vi "Initialize DLL Readers.vi"(8 "error in (no error)":errorcluster, 10 "Poll Timeout [5 ms]":i32=5, 11 "Phasor Data Concentrator in":refnum<class "Phasor Data Concentrator.lvclass">) -> (0 "error out":errorcluster, 3 "Phasor Data Concentrator out":refnum<class "Phasor Data Concentrator.lvclass">)   [LabVIEW 2013, in "PMU Recorder Light.lvlib" / "Phasor Data Concentrator.lvclass"]
uses:
  Phasor Data Concentrator.lvclass
  Phasor Data Concentrator.lvclass/Phasor Data Concentrator.ctl
  PMU Recorder Light.lvlib
  Statnett C37.118 DLL/Statnett C37.118 DLL.lvclass
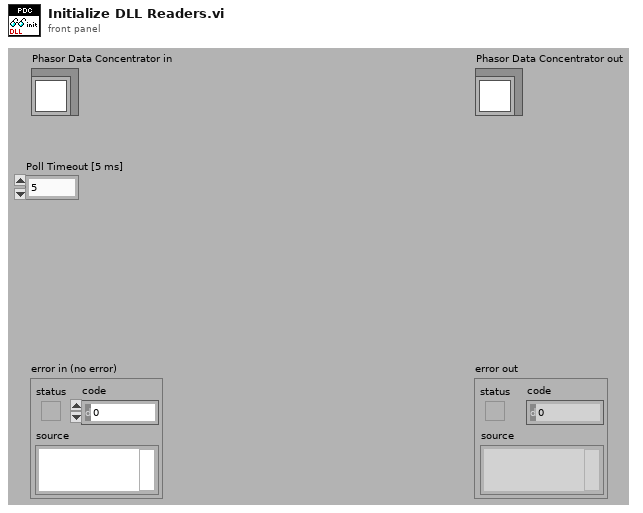
[diagram p1: front panel]
types:
  T1 = cluster{"Phasor":string[], "Analog":string[], "Digital":string[]}
  T2 = cluster{"Pseudo PDC ID":i32, cluster{i32, i32, i32}}
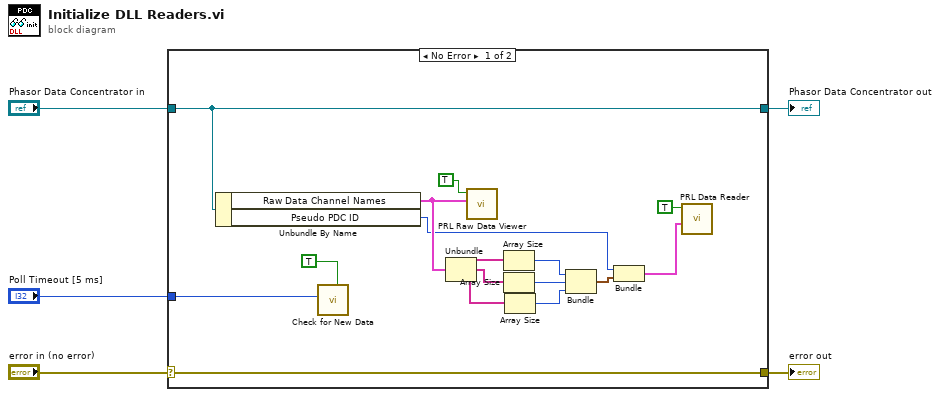
[diagram p0: block diagram]
diagram:
  n1 = case shown="No Error" "error in (no error)" {
    selector: "error in (no error)" -> [w21 w23]
    tunnel: [w21 w23] -> w4
    tunnel: [w20 w22] -> w2
    tunnel: "Phasor Data Concentrator in" -> [w20 w22]
    tunnel: "Poll Timeout [5 ms]" -> [w6 _]
    frame No Error {
      n2 = Unbundle By Name(w20) -> ("Raw Data Channel Names"=w17:T1, "Pseudo PDC ID"=w9:i32)
      n3 = call "Check for New Data.vi"("Set Timeout"=TRUE, "Poll Timeout [5 ms]"=w6) -> ()  [unwired: 8 in, 2 out]
      n4 = Unbundle(w17) -> ("Phasor"=w16:string[], "Analog"=w15:string[], "Digital"=w14:string[])
      n5 = call "PRL Raw Data Viewer.vi"("Raw Data Channel Names"=w17, "Initialize"=TRUE) -> ()  [unwired: 10 in]
      n6 = Array Size(array=w16) -> (size(s)=w13:i32)
      n7 = Array Size(array=w15) -> (size(s)=w12:i32)
      n8 = Array Size(array=w14) -> (size(s)=w11:i32)
      n9 = Bundle(w13, w12, w11) -> (w10:cluster{i32, i32, i32})  [unwired: 1 in]
      n10 = Bundle("Pseudo PDC ID"=w9, w10) -> (w8:T2)  [unwired: 1 in]
      n11 = call "PRL Data Reader.vi"("Initialize Data"=w8, "Initialize"=TRUE) -> ()  [unwired: 3 in, 7 out]
    }
    frame Error {
    }
  }
  "error out" <- w4
  "Phasor Data Concentrator out" <- w2
